vi "Save Data File.vi"(8 "error in (no error)":errorcluster, 9 "Open File Location":bool, 10 "Data":dbl[](array[numeric]), 11 "File Type":T1) -> (0 "error out":errorcluster)   [LabVIEW 2020]
uses:
  Controls/File Type.ctl
  <vilib>/Utility/TDMS File Viewer/NI_TDMS File Viewer.lvlib
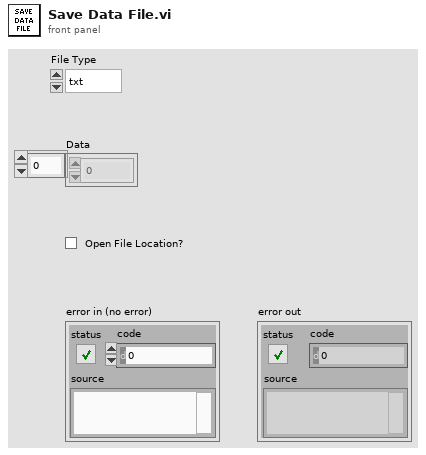
[diagram p1: front panel]
types:
  T1 = typedef "File Type.ctl" = enum16{"txt", "csv", "tdms"}
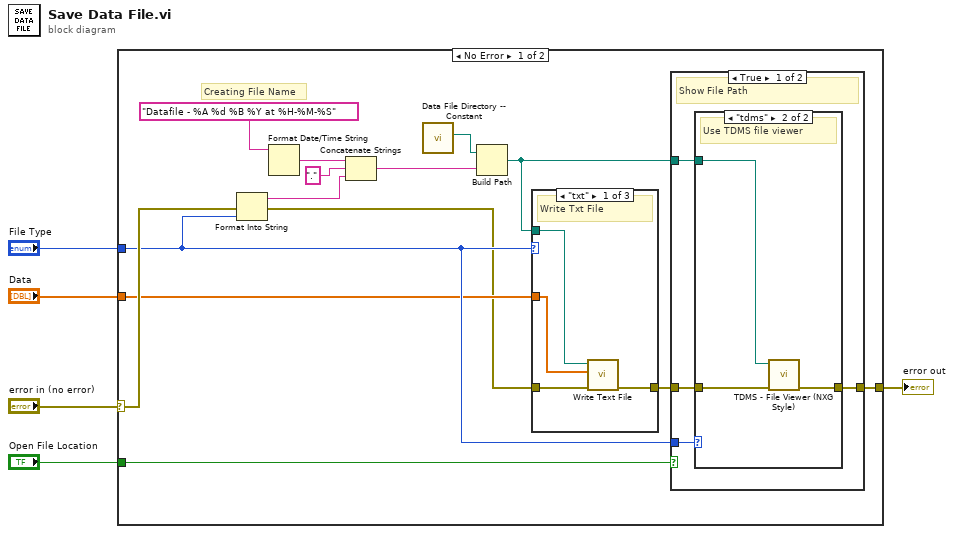
[diagram p0: block diagram]
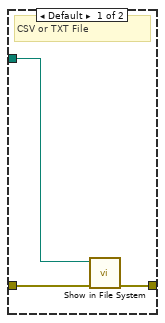
[diagram p2: hidden frame]
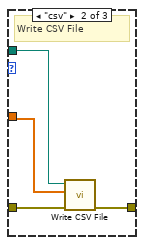
[diagram p4: hidden frame]
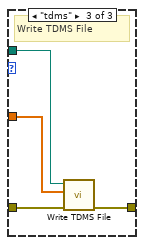
[diagram p5: hidden frame]
diagram:
  n1 = case shown="No Error" "error in (no error)" {
    selector: "error in (no error)" -> [w19 w43]
    tunnel: "File Type" -> [w12 _]
    tunnel: "Open File Location" -> [w13 _]
    tunnel: [w8 w43] -> w2
    tunnel: "Data" -> [w11 _]
    frame No Error {
      # "Creating File Name"
      n2 = Format Into String(error in=w19, w12) -> (resulting string=w16:string, error out=w10:errorcluster)  [unwired: 2 in]
      n3 = Format Date/Time String(time format string (%c)="Datafile - %A %d %B %Y at %H-%M-%S" ("format string")) -> (date/time string=w17:string)  [unwired: 2 in]
      n4 = Concatenate Strings(w17, "." ("string"), w16) -> (w14:string)
      n5 = call "Data File Directory -- Constant.vi"() -> ("Data File Directory"=w6:path)  [unwired: 11 in]
      n6 = Build Path(base path=w6, name or relative path=w14) -> (appended path=w7:path)
      n7 = case shown="\"txt\"" w12 {
        tunnel: w7 -> [w32 w38 w41]
        tunnel: w11 -> [w31 w35 w42]
        tunnel: w10 -> [w34 w37 w40]
        tunnel: [w33 w36 w39] -> w9
        frame "txt" {
          # "Write Txt File"
          n8 = call "Write Text File.vi"("error in (no error)"=w34, "Data"=w31, "Path"=w32) -> ("error out"=w33:errorcluster)  [unwired: 8 in]
        }
        frame "csv" {
          # "Write CSV File"
          n9 = call "Write CSV File.vi"("error in (no error)"=w37, "Data"=w35, "Path"=w38) -> ("error out"=w36:errorcluster)  [unwired: 8 in]
        }
        frame "tdms" {
          # "Write TDMS File"
          n10 = call "Write TDMS File.vi"("error in (no error)"=w40, "Data"=w42, "Path"=w41) -> ("error out"=w39:errorcluster)  [unwired: 8 in]
        }
      }
      n11 = case shown="True" w13 {
        tunnel: w12 -> [w23 _]
        tunnel: w9 -> [w22 w30]
        tunnel: [w21 w30] -> w8
        tunnel: w7 -> [w20 _]
        frame True {
          # "Show File Path"
          n12 = case shown="\"tdms\"" w23 {
            tunnel: w22 -> [w25 w28]
            tunnel: [w24 w27] -> w21
            tunnel: w20 -> [w26 w29]
            frame Default {
              # "CSV or TXT File"
              n13 = call <vilib>:"Show in File System.vi"("error in (no error)"=w25, "file or directory path"=w26) -> ("error out"=w24:errorcluster)  [unwired: 9 in]
            }
            frame "tdms" {
              # "Use TDMS file viewer"
              n14 = call <vilib>:"TDMS - File Viewer (NXG Style).vi"("error in"=w28, "file in"=w29) -> ("error out"=w27:errorcluster)  [unwired: 8 in, 1 out]
            }
          }
        }
        frame False {
          # "Don't Show File Path"
        }
      }
    }
    frame Error {
    }
  }
  "error out" <- w2
